vi "JKISM++ Global Log Event.vi"(8 "Error in":errorcluster caption="Error in (no error)") -> (0 "Error out":errorcluster, 3 "JKISM Global Log Event":refnum<user-event>)   [LabVIEW 2014, in "JKI-State-Machine-Plus.lvlib"]
uses:
  JKI-State-Machine-Plus.lvlib
  _Support/Typedef/_JKI StateMachine Current State.ctl
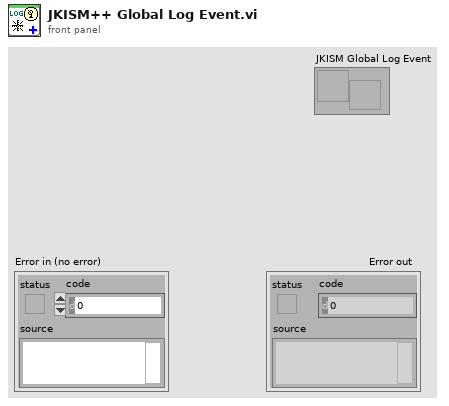
[diagram p1: front panel]
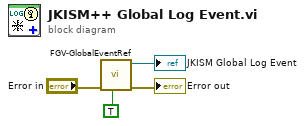
[diagram p0: block diagram]
diagram:
  n1 = call "FGV-GlobalEventRef.vi"("Create(F)"=TRUE, "error in (no error)"="Error in") -> ("error out"=→"Error out":errorcluster, "JKISM Global Log Event"=→"JKISM Global Log Event":refnum<user-event>)  [unwired: 8 in]
